vi "pixie divide peak height.vi"(0 "channel 0":u16[](array[numeric]), 1 "size of array":i16, 5 "channel 1":u16[](array[numeric]), 7 "channel 2":u16[](array[numeric]), 9 "channel 3":u16[](array[numeric]), 11 "error in (no error)":errorcluster, 12 "scale factor":u32=2) -> (4 "output channel 0-3":u32[][](array[numeric]), 15 "error out":errorcluster)   [LabVIEW 2016]
doc: "Takes values from pixie and divides each channel by a fixed value.\nThis is used to insure the spectrum fits inside a 1024x1024 array"
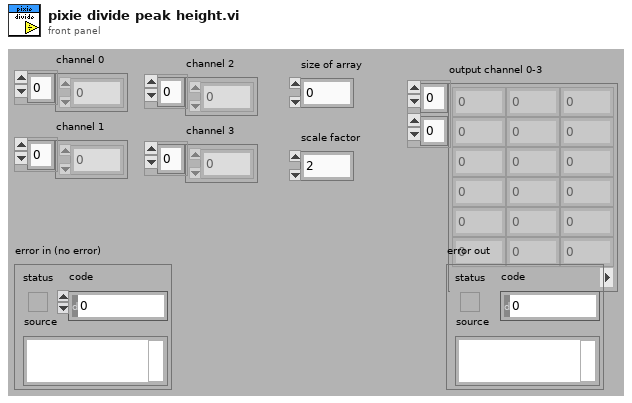
[diagram p1: front panel]
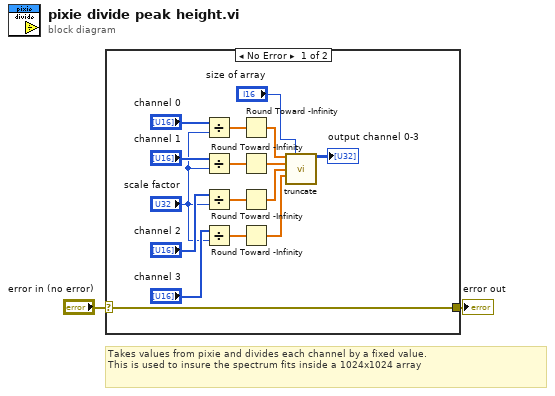
[diagram p0: block diagram]
diagram:
  # "Takes values from pixie and divides each channel by a fixed value.\nThis is used to insure the spectrum fits inside a 1024x1024 array"
  n1 = case shown="No Error" "error in (no error)" {
    selector: "error in (no error)" -> [w3 w19]
    tunnel: [w3 w19] -> w1
    frame No Error {
      n2 = Divide(x="channel 0", y="scale factor") -> (x/y=w4:dbl[])
      n3 = Divide(x="channel 1", y="scale factor") -> (x/y=w5:dbl[])
      n4 = Divide(x="channel 2", y="scale factor") -> (x/y=w6:dbl[])
      n5 = Divide(x="channel 3", y="scale factor") -> (x/y=w7:dbl[])
      n6 = Round Toward -Infinity(1:w4) -> (0:w9:dbl[])
      n7 = Round Toward -Infinity(1:w5) -> (0:w10:dbl[])
      n8 = Round Toward -Infinity(1:w6) -> (0:w11:dbl[])
      n9 = Round Toward -Infinity(1:w7) -> (0:w12:dbl[])
      n10 = call "truncate.vi"("input array 0"=w9, "size of array"="size of array", "input array 1"=w10, "input array 2"=w11, "input array 3"=w12) -> ("output channel 0-3"=→"output channel 0-3":u32[][])  [unwired: 9 in, 1 out]
    }
    frame Error {
    }
  }
  "error out" <- w1
